vi "AcquireHardware.vi"(8 "error in (no error)":errorcluster, 11 "PCO in":refnum<class "PCO_Camera.lvclass">) -> (0 "error out":errorcluster, 2 "Image Out":T1(plugin-control), 3 "PCO out":refnum<class "PCO_Camera.lvclass">)   [LabVIEW 2020, in "PCO_Camera.lvclass"]
uses:
  PCO_Camera.lvclass
  C:/GEECS/Developers Version/source/Device Drivers/Point Grey Camera/Point Grey Camera.lvclass
  Point Grey Camera/Point Grey Camera.lvclass/Point Grey Camera.ctl
  PCO_Camera.lvclass/PCO_Camera.ctl
  Point Grey Camera/Read Image ref.vi
  Point Grey Camera/Read Settings 2.vi
  pco.labview/pco.camera/Camera.lvclass
  pco.labview/pco.sdk/TimingControl/TimingControl.lvlib
panel:
  out "acq time (ms)":u32
  out "Intensity Graph Mono":u16[][](graph)
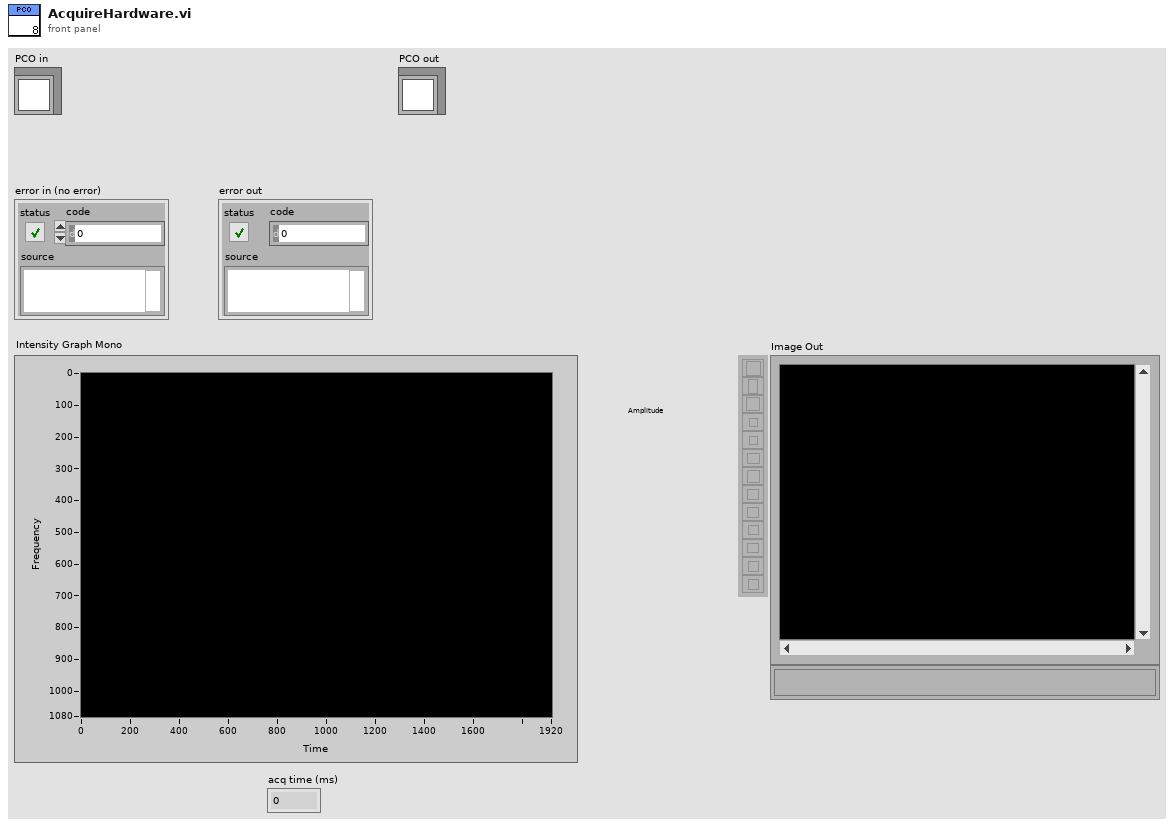
[diagram p1: front panel]
types:
  T1 = typedef "IMAQ Image.ctl" = refnum<image>
  T2 = typedef "Point Grey Camera.lvclass/SettingsTypdef.ctl" = cluster{"Trigger":T3, "Gain":cluster{"Value":dbl, "Min":dbl, "Max":dbl, "StepSize":dbl, "Tolerance":dbl, "valueactual":dbl}, "Exposure":cluster{"Value":dbl, "Min":dbl, "Max":dbl, "StepSize":dbl, "Tolerance":dbl, "valueactual":dbl}, "Timeout":cluster{"Value":dbl, "Min":dbl, "Max":dbl, "StepSize":dbl, "Tolerance":dbl, "valueactual":dbl}, "LocalSavingPath":path, "Save":T3, "TriggerDelay":cluster{"Value":dbl, "Min":dbl, "Max":dbl, "StepSize":dbl, "Tolerance":dbl, "valueactual":dbl}, "CamSession":string, "ROI":T4, "MaxGUIPixel":cluster{"Value":dbl, "Min":dbl, "Max":dbl, "StepSize":dbl, "Tolerance":dbl, "valueactual":dbl}, "Target":cluster{"X":cluster{"Value":dbl, "Min":dbl, "Max":dbl, "StepSize":dbl, "Tolerance":dbl, "valueactual":dbl}, "Y":cluster{"Value":dbl, "Min":dbl, "Max":dbl, "StepSize":dbl, "Tolerance":dbl, "valueactual":dbl}}, "Analysis":T3, "maxshot#":dbl, "SpatialCalibration":cluster{"Value":dbl, "Min":dbl, "Max":dbl, "StepSize":dbl, "Tolerance":dbl, "valueactual":dbl}, "roistatus":T3, "Lineout":T3, "AnalysisThreshold":cluster{"Value":dbl, "Min":dbl, "Max":dbl, "StepSize":dbl, "Tolerance":dbl, "valueactual":dbl}, "TargetSize":cluster{"X":cluster{"Value":dbl, "Min":dbl, "Max":dbl, "StepSize":dbl, "Tolerance":dbl, "valueactual":dbl}, "Y":cluster{"Value":dbl, "Min":dbl, "Max":dbl, "StepSize":dbl, "Tolerance":dbl, "valueactual":dbl}}, "Simulation":T3, "SpatialCalibrationY":cluster{"Value":dbl, "Min":dbl, "Max":dbl, "StepSize":dbl, "Tolerance":dbl, "valueactual":dbl}, "Target2":cluster{"X":cluster{"Value":dbl, "Min":dbl, "Max":dbl, "StepSize":dbl, "Tolerance":dbl, "valueactual":dbl}, "Y":cluster{"Value":dbl, "Min":dbl, "Max":dbl, "StepSize":dbl, "Tolerance":dbl, "valueactual":dbl}}, "Target2Size":cluster{"X":cluster{"Value":dbl, "Min":dbl, "Max":dbl, "StepSize":dbl, "Tolerance":dbl, "valueactual":dbl}, "Y":cluster{"Value":dbl, "Min":dbl, "Max":dbl, "StepSize":dbl, "Tolerance":dbl, "valueactual":dbl}}, "Crosshair":cluster{"Label1":string, "Label2":string}, "Max2ndMomRadius":cluster{"Value":dbl, "Min":dbl, "Max":dbl, "StepSize":dbl, "Tolerance":dbl, "valueactual":dbl}, "SaveType":T5, "BackgroundPath":path, "GUI8bit":T3, "GUICompression":T3, "CompressionQuality":cluster{"Value":dbl, "Min":dbl, "Max":dbl, "StepSize":dbl, "Tolerance":dbl, "valueactual":dbl}, "SaveAsync":T3, "PerspectivePath":path, "PerspectiveCorrectGUI":T3, "BlackLevel":cluster{"Value":dbl, "Min":dbl, "Max":dbl, "StepSize":dbl, "Tolerance":dbl, "valueactual":dbl}, "TargetBP":cluster{"X":cluster{"Value":dbl, "Min":dbl, "Max":dbl, "StepSize":dbl, "Tolerance":dbl, "valueactual":dbl}, "Y":cluster{"Value":dbl, "Min":dbl, "Max":dbl, "StepSize":dbl, "Tolerance":dbl, "valueactual":dbl}}, "PythonAnalysis":T3, "PythonFunctionName":string, "PythonLineout":T3, "PythonVersion":string, "GEECSBuildsPath":path, "DisplayPythonProcessedImage":T3, "PythonModuleName":string, "AnalysisThresholdHigh":cluster{"Value":dbl, "Min":dbl, "Max":dbl, "StepSize":dbl, "Tolerance":dbl, "valueactual":dbl}, "AnalysisMedianRank":cluster{"Value":dbl, "Min":dbl, "Max":dbl, "StepSize":dbl, "Tolerance":dbl, "valueactual":dbl}, "ClockSpeed":cluster{"Value":dbl, "Min":dbl, "Max":dbl, "StepSize":dbl, "Tolerance":dbl, "valueactual":dbl}, "AutoTrigger":T3, "AutoTriggerLevelMeanCounts":cluster{"Value":dbl, "Min":dbl, "Max":dbl, "StepSize":dbl, "Tolerance":dbl, "valueactual":dbl}, "AnalysisROILeft":cluster{"Value":dbl, "Min":dbl, "Max":dbl, "StepSize":dbl, "Tolerance":dbl, "valueactual":dbl}, "AnalysisROIRight":cluster{"Value":dbl, "Min":dbl, "Max":dbl, "StepSize":dbl, "Tolerance":dbl, "valueactual":dbl}, "AnalysisROITop":cluster{"Value":dbl, "Min":dbl, "Max":dbl, "StepSize":dbl, "Tolerance":dbl, "valueactual":dbl}, "AnalysisROIBottom":cluster{"Value":dbl, "Min":dbl, "Max":dbl, "StepSize":dbl, "Tolerance":dbl, "valueactual":dbl}, "AnalysisROI":T3, "UseSoftwareTrigger":T3, "UDPtrigger":T3, "AutoTriggerLevelMaxCounts":cluster{"Value":dbl, "Min":dbl, "Max":dbl, "StepSize":dbl, "Tolerance":dbl, "valueactual":dbl}}
  T3 = typedef "OnOffTypeDef.ctl" = enum16{"off", "on"}
  T4 = typedef "ROI_TypDef.ctl" = cluster{"Width":cluster{"Value":dbl, "Min":dbl, "Max":dbl, "StepSize":dbl, "Tolerance":dbl, "valueactual":dbl}, "Height":cluster{"Value":dbl, "Min":dbl, "Max":dbl, "StepSize":dbl, "Tolerance":dbl, "valueactual":dbl}, "OffsetX":cluster{"Value":dbl, "Min":dbl, "Max":dbl, "StepSize":dbl, "Tolerance":dbl, "valueactual":dbl}, "OffsetY":cluster{"Value":dbl, "Min":dbl, "Max":dbl, "StepSize":dbl, "Tolerance":dbl, "valueactual":dbl}}
  T5 = typedef "Image save type.ctl" = enum16{"PNG", "BMP", "JPEG", "TDMS", "hdf5"}
  T6 = enum16{"Undefined", "Mono8", "Mono16", "BGRA8", "RGBA8", "BGRA16", "RGBA16", "CompressedMono8"}
  T7 = typedef "Camera.lvclass/binning.ctl" = cluster{"vert":u16, "horz":u16}
  T8 = cluster{"exposure_time_s":dbl, "delay_time_s":dbl, "roi":cluster{"x0":u64, "y0":u64, "x1":u64, "y1":u64}, "timestamp_mode":u16, "pixelrate":u32, "trigger_mode":u16, "acquire_mode":u16, "metadata_mode":u16, "noisefilter_mode":u16, "binning":T7}
  T9 = cluster{"dwImgCounter":u32, "lvTimestamp":timestamp, "dwMicroSeconds":u32}
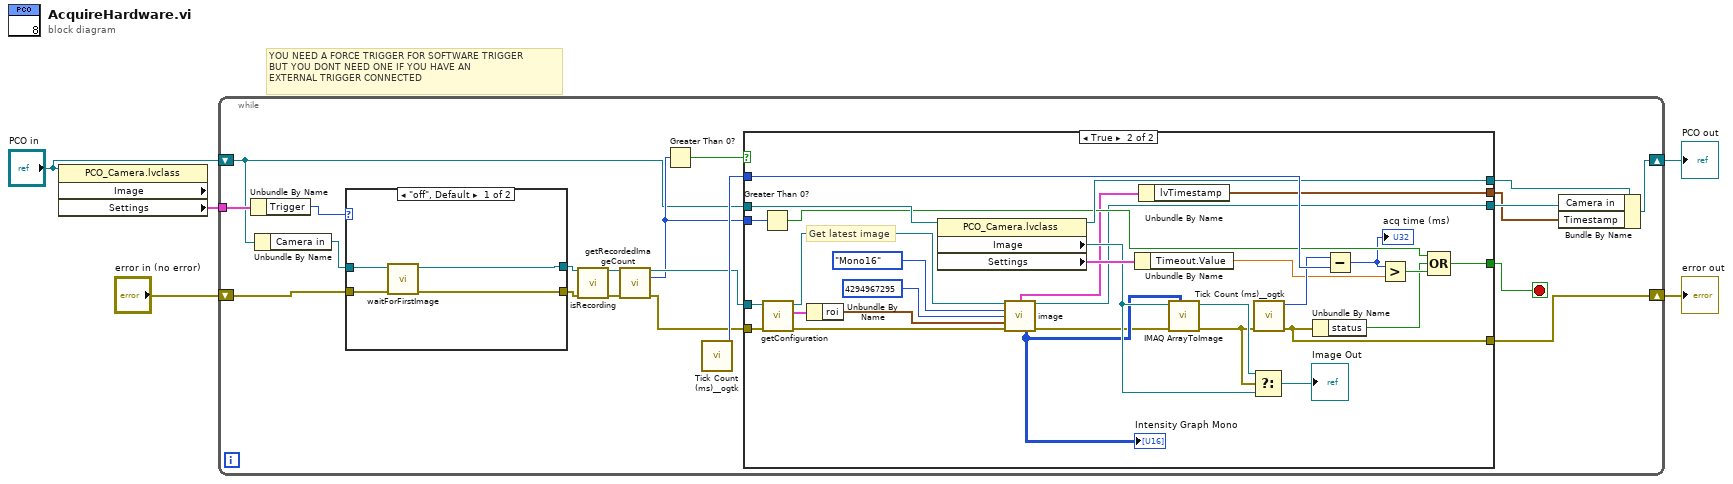
[diagram p0: block diagram]
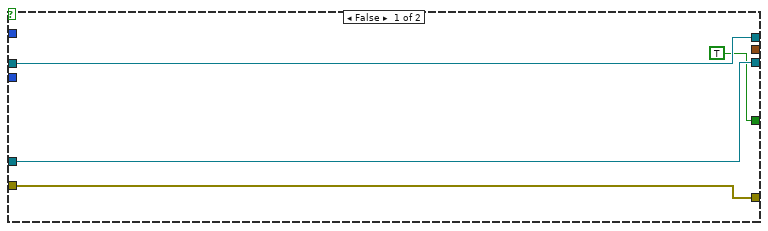
[diagram p2: hidden frame]
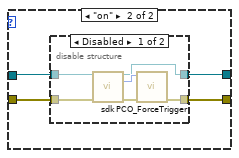
[diagram p3: hidden frame]
diagram:
  # "YOU NEED A FORCE TRIGGER FOR SOFTWARE TRIGGER \nBUT YOU DONT NEED ONE IF YOU HAVE AN \nEXTERNAL TRIGGER CONNECTED"
  n1 = property class="PCO_Camera.lvclass" props=["Image", "Settings"](reference="PCO in") -> ("Settings"=w2:T2)  [unwired: 1 in, 3 out]
  n2 = while {
    tunnel: w2 -> [w23]
    shift-right: [w14] -> w5
    shift-left: "PCO in" -> [w8]
    shift-right: [w24] -> w4
    shift-left: "error in (no error)" -> [w21]
    stop <- w18 stop-if-true
    n3 = Unbundle By Name(w23) -> ("Trigger"=w22:T3)
    n4 = Unbundle By Name(w8) -> ("Camera in"=w7:refnum<class "Camera.lvclass">)
    n5 = case shown="\"off\", Default" w22 {
      tunnel: [w63 w67] -> w12
      tunnel: [w62 w66] -> w11
      tunnel: w21 -> [w61 w65]
      tunnel: w7 -> [w60 w64]
      frame "off", Default {
        n6 = call-dynamic "waitForFirstImage.vi"("error in (no error)"=w61, "Camera in"=w60) -> ("error out"=w62:errorcluster, "Camera out"=w63:refnum<class "Camera.lvclass">)  [unwired: 8 in]
      }
      frame "on" {
        n7 = disable-structure shown="Disabled" {
          disable-tunnel: [w71 w74] -> w67
          disable-tunnel: [w70 w75] -> w66
          disable-tunnel: w64 -> [w69 w74]
          disable-tunnel: w65 -> [w68 w75]
          frame Disabled {
            n8 = call-dynamic "sdk.vi"("Camera in"=w69, "error in (no error)"=w68) -> ("Camera out"=w71:refnum<class "Camera.lvclass">, "sdk"=w73:u64, "error out"=w72:errorcluster)  [unwired: 11 in]
            n9 = call "PCO_ForceTrigger.vi"("error in (no error)"=w72, "ph"=w73) -> ("error out"=w70:errorcluster)  [unwired: 6 in, 3 out]
          }
          frame Enabled {
          }
        }
      }
    }
    n10 = call-dynamic "isRecording.vi"("Camera in"=w12, "error in (no error)"=w11) -> ("Camera out"=w10:refnum<class "Camera.lvclass">, "error out"=w9:errorcluster)  [unwired: 11 in, 1 out]
    n11 = call-dynamic "getRecordedImageCount.vi"("Camera in"=w10, "error in (no error)"=w9) -> ("Camera out"=w20:refnum<class "Camera.lvclass">, "recorded_image_count"=w16:u32, "error out"=w19:errorcluster)  [unwired: 11 in]
    n12 = Greater Than 0?(x=w16) -> (x > 0?=w17:bool)
    n13 = call <userlib>:"Tick Count (ms)__ogtk.vi"() -> ("millisecond timer value"=w25:u32)  [unwired: 10 in, 1 out]
    n14 = case shown="True" w17 {
      tunnel: w25 -> [_ w59]
      tunnel: [w29 w58] -> w15
      tunnel: [w28 w57] -> w24
      tunnel: w8 -> [w29 w56]
      tunnel: w20 -> [w27 w46]
      tunnel: w16 -> [_ w40]
      tunnel: w19 -> [w28 w36]
      tunnel: [TRUE w33] -> w18
      tunnel: [w27 w32] -> w13
      tunnel: [_ w30] -> w6
      frame False {
      }
      frame True {
        # "Get latest image"
        n15 = Greater Than 0?(x=w40) -> (x > 0?=w38:bool)
        n16 = call-dynamic "getConfiguration.vi"("error in (no error)"=w36, "Camera in"=w46) -> ("error out"=w35:errorcluster, "configuration"=w53:T8, "Camera out"=w51:refnum<class "Camera.lvclass">)  [unwired: 7 in]
        n17 = Unbundle By Name(w53) -> ("roi"=w52:cluster{"x0":u64, "y0":u64, "x1":u64, "y1":u64})
        n18 = property class="PCO_Camera.lvclass"(reference=w56) -> (reference out=w58:refnum<class "PCO_Camera.lvclass">, "Image"=w48:T1, "Settings"=w50:T2)  [unwired: 1 in, 1 out]
        n19 = call-dynamic "image.vi"("Camera in"=w51, "data_format"=T6."Mono16", "image_index"=u32 4294967295 ("dwImgIdx"), "roi"=w52, "error in (no error)"=w35) -> ("timestamp"=w31:T9, "Camera out"=w32:refnum<class "Camera.lvclass">, "raw_image (U16)"=w39:u16[][], "error out"=w34:errorcluster)  [unwired: 3 in, 4 out]
        "Intensity Graph Mono" <- w39
        n20 = Unbundle By Name(w50) -> ("Timeout.Value"=w43:dbl)
        n21 = Unbundle By Name(w31) -> ("lvTimestamp"=w30:timestamp)
        n22 = call "IMAQ ArrayToImage"("Image Pixels (U16)"=w39, "error in (no error)"=w34, "Image"=w48) -> ("error out"=w45:errorcluster, "Image Out"=w49:T1)  [unwired: 7 in]
        n23 = Select(t=w49, s=w45, f=w48) -> (s? t:f=→"Image Out":T1)
        n24 = call <userlib>:"Tick Count (ms)__ogtk.vi"("error in (no error)"=w45) -> ("error out"=w57:errorcluster, "millisecond timer value"=w44:u32)  [unwired: 9 in]
        n25 = Unbundle By Name(w57) -> ("status"=w41:bool)
        n26 = Subtract(x=w44, y=w59) -> (x-y=w37:u32)
        "acq time (ms)" <- w37
        n27 = Greater?(x=w37, y=w43) -> (0:w42:bool)
        n28 = Compound Arithmetic op=OR(w38, w41, w42) -> (w33:bool)
      }
    }
    n29 = Bundle By Name(cluster=w15, "Camera in"=w13, "Timestamp"=w6) -> (w14:refnum<class "PCO_Camera.lvclass">)
  }
  "error out" <- w4
  "PCO out" <- w5
